vi "S2C_SetExeLoop.vi"(8 "Error In":errorcluster, 11 "MenuRef":refnum<k9>) -> (0 "Error Out":errorcluster)   [LabVIEW 2015]
doc: "Toggles the \"Local File\" runtime menu item."
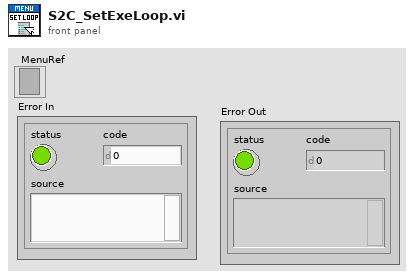
[diagram p1: front panel]
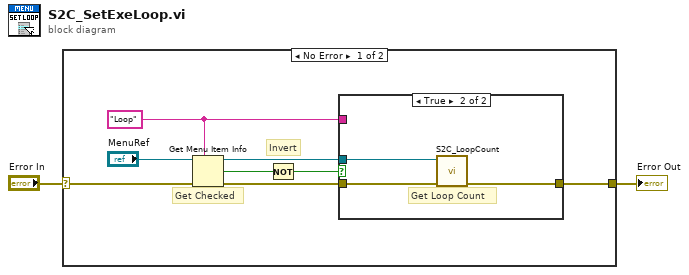
[diagram p0: block diagram]
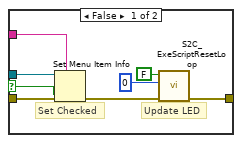
[diagram p2: hidden frame]
diagram:
  n1 = case shown="No Error" "Error In" {
    selector: "Error In" -> [w10 w22]
    tunnel: [w3 w22] -> w1
    frame No Error {
      w8 = "Loop" ("item tag")
      # "Invert"
      # "Get Checked"
      n2 = Get Menu Item Info(7:w8, 8:w10, 11:"MenuRef") -> (0:w7:errorcluster, 3:w6:refnum<k9>, 4:w5:bool)  [unwired: 4 out]
      n3 = Not(x=w5) -> (.not. x?=w4:bool)
      n4 = case shown="True" w4 {
        selector: w4 -> [w11 _]
        tunnel: w8 -> [w18 _]
        tunnel: w7 -> [w17 w21]
        tunnel: w6 -> [w16 w19]
        tunnel: [w13 w20] -> w3
        frame False {
          # "Update LED"
          # "Set Checked"
          n5 = Set Menu Item Info(6:w11, 7:w18, 8:w17, 11:w16) -> (0:w14:errorcluster)  [unwired: 3 in, 1 out]
          n6 = call "S2C_ExeScriptResetLoop.vi"("Error In"=w14, "Loops"=0, "Loop?"=FALSE) -> ("Error Out"=w13:errorcluster)  [unwired: 8 in]
        }
        frame True {
          # "Get Loop Count"
          n7 = call "S2C_LoopCount.vi"("Error In"=w21, "MenuRef"=w19) -> ("Error Out"=w20:errorcluster)  [unwired: 9 in]
        }
      }
    }
    frame Error {
    }
  }
  "Error Out" <- w1
